vi "SPI_SetMode.vi"(5 "Device":i32, 6 "Mode":u8 format="%02b", 7 "Bus":i32=1, 8 "error in":errorcluster) -> (0 "error out":errorcluster)   [LabVIEW 2014]
doc: "Select the SPI mode for the current device. Mode is a two-bit value (0-3), the MSB determines the clock polarity and the LSB determines the phase."
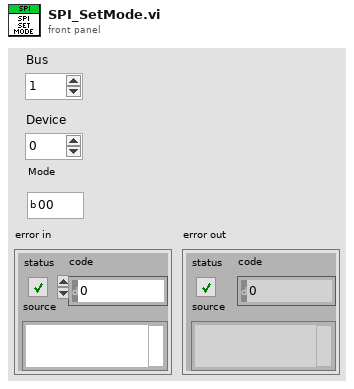
[diagram p1: front panel]
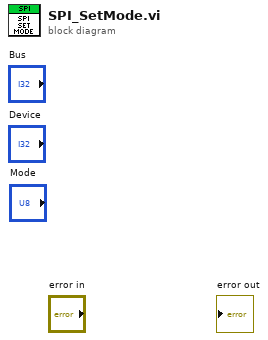
[diagram p0: block diagram]
diagram:
